vi "Robot Main.vi"() -> ()   [LabVIEW 2013]
doc: "This VI imlements the framework and scheduler for your robotics program. It should not be necessary to modify the framework. You are expected to add your code to the VIs called from Robot Main, the ones located in the Team Code within the project."
uses:
  Command Type.ctl
panel:
  in  "Update":bool
  in  "Functions":string
  in  "Finish":bool
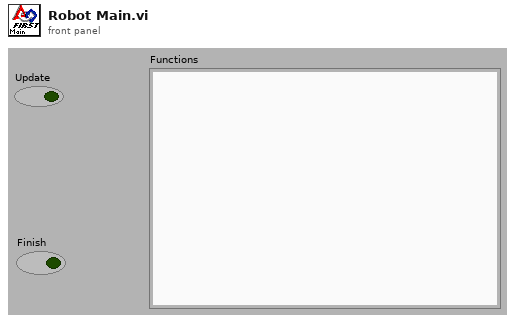
[diagram p1: front panel]
types:
  T1 = typedef "Command Type.ctl" = cluster{"Function Name":string, "Arguments":string[]}
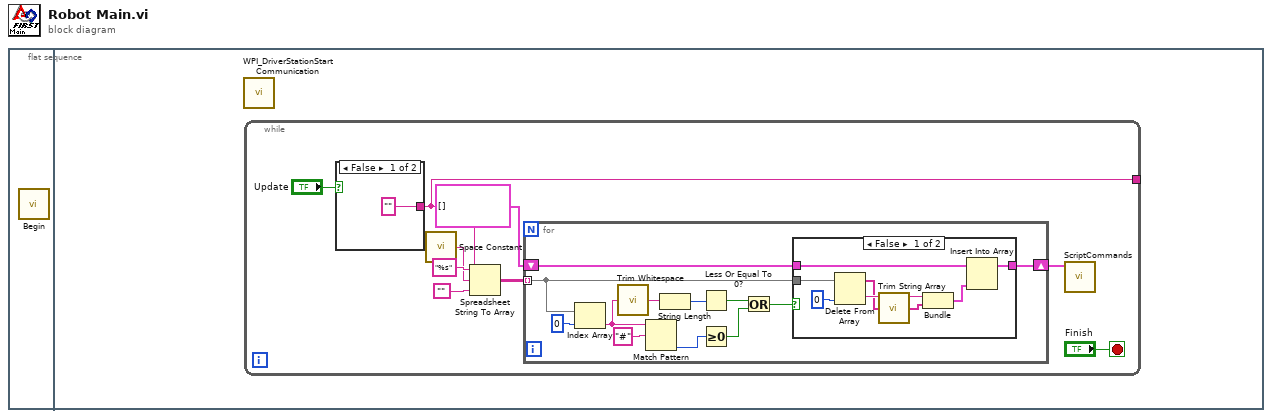
[diagram p0: block diagram]
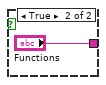
[diagram p2: hidden frame]
diagram:
  n1 = flat-sequence {
    frame #0 {
      n2 = call "Begin.vi"() -> ()  [unwired: 12 in]
    }
    frame #1 {
      n3 = call <vilib>:"WPI_DriverStationStart Communication.vi"() -> ()  [unwired: 1 in, 11 out]
      n4 = while {
        tunnel: [w2] -> _
        stop <- "Finish" stop-if-true
        n5 = case shown="False" "Update" {
          tunnel: ["" "Functions"] -> w2
          frame False {
          }
          frame True {
          }
        }
        n6 = call <vilib>:"Space Constant.vi"() -> ("String"=w7:string)
        n7 = Spreadsheet String To Array(delimiter (Tab)=w7, format string="%s", spreadsheet string=w2, array type (2D Dbl)="") -> (array=w6:string[][])
        n8 = for {
          tunnel: w6 -> [w13] mode=indexing
          shift-right: [w14] -> w1
          shift-left: T1[] [] ("Auton Routine") -> [w21]
          n9 = Index Array(array=w13, index=0) -> (element=w18:string)
          n10 = call <vilib>:"Trim Whitespace.vi"("string"=w18) -> ("trimmed string"=w12:string)  [unwired: 1 in]
          n11 = Match Pattern(string=w18, regular expression="#") -> (offset past match=w20:i32)  [unwired: 1 in, 3 out]
          n12 = String Length(string=w12) -> (length=w19:i32)
          n13 = Less Or Equal To 0?(x=w19) -> (x <= 0?=w15:bool)
          n14 = Greater Or Equal To 0?(x=w20) -> (x >= 0?=w16:bool)
          n15 = Or(x=w15, y=w16) -> (x .or. y?=w17:bool)
          n16 = case shown="False" w17 {
            tunnel: w21 -> [w28 w32]
            tunnel: [w27 w32] -> w14
            tunnel: w13 -> [w31 _]
            frame False {
              n17 = Delete From Array(array=w31, index=0) -> (deleted portion=w29:string, array with subset deleted=w26:string[])  [unwired: 1 in]
              n18 = call "Trim String Array.vi"("String Array"=w26) -> ("String Array Trimmed"=w25:string[])  [unwired: 14 in]
              n19 = Bundle(w29, "String Array Trimmed"=w25) -> (w24:cluster{string, "String Array Trimmed":string[]})  [unwired: 1 in]
              n20 = Insert Into Array(array=w28, new element=w24) -> (w27:T1[])  [unwired: 1 in]
            }
            frame True {
            }
          }
        }
        n21 = call "ScriptCommands.vi"("Auton Routines"=w1) -> ()  [unwired: 11 in]
      }
    }
  }
